vi "SQLite Operation Tests.vi"   [LabVIEW 2023]
uses:
  <vilib>/addons/_JKI Toolkits/Caraya/classes/Test/Test.lvclass
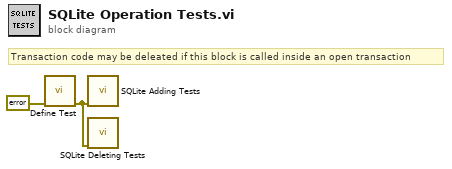
[diagram p0: block diagram]
diagram:
  # "Transaction code may be deleated if this block is called inside an open transaction"
  n1 = call <vilib>:"Define Test.vi"("error in (no error)"=errorcluster {"status"=FALSE, "code"=0, "source"=""}) -> ("error out"=w1:errorcluster)  [unwired: 9 in, 1 out]
  n2 = call "SQLite Adding Tests.vi"("Error In (no error)"=w1) -> ()  [unwired: 10 in, 1 out]
  n3 = call "SQLite Deleting Tests.vi"("Error In (no error)"=w1) -> ()  [unwired: 10 in, 1 out]
